vi "Diagnostics.vi"(10 "Parameters":variant, 11 "Process":refnum<class "Process.lvclass">) -> ()   [LabVIEW 2019, in "Diagnostics Addon Engine.lvlib"]
uses:
  Diagnostics Addon Engine.lvlib
  <vilib>/NI/NIVS Inline Async API/_VS Inline Async API/Process/Process.lvclass
  Addon Shared/Types/SysDef.Compile.ctl
  Addon Shared/Types/CAN.ctl
  Addon Shared/Types/CAN.Interface.ctl
  Addon Shared/Types/Protocol.ctl
  Addon Shared/Types/Transport.ctl
  Addon Shared/Types/986x.ctl
  Addon Shared/Types/Frame.Compile.ctl
  Addon Shared/Types/Type.ctl
  Addon Shared/Types/Signal.ctl
  Addon Shared/Types/DPID.ctl
  Addon Shared/Types/DPID.Rate.ctl
  Addon Shared/Types/DTC.Settings.ctl
  Addon Shared/Types/DTC.Descriptor.ctl
  Addon Shared/Types/Poll.Compiled.ctl
  Addon Shared/Types/Security.ctl
  Addon Shared/Types/Security.Type.ctl
  <vilib>/NI/NIVS Inline Async API/_Data Access Engine/Access Type Classes/Write/Write.lvclass/Write.ctl
  <vilib>/NI/NIVS Inline Async API/_Data Access Engine/Access Type Classes/ReadWrite/ReadWrite.lvclass/ReadWrite.ctl
  <vilib>/NI/NI VeriStand Addon Network Comm/Engine/VeriStand Comm.lvclass/VeriStand Comm.ctl
  <vilib>/NI/NIVS Inline Async API/_Data Access Engine/Access Type Classes/Read/Read.lvclass/Read.ctl
  <vilib>/NI/NIVS Inline Async API/_VS Inline Async API/Process/Process.lvclass/Process.ctl
  SubVIs/Frames.Refs.Cleanup.vi
  <vilib>/NI/NIVS Inline Async API/_Data Access Engine/Data Access Engine/Methods/Data.Processes.Execute.vi
  <vilib>/NI/NIVS Inline Async API/_Data Access Engine/Data Access Engine/Methods/Write.Data.vi
  <vilib>/NI/NI VeriStand Addon Network Comm/Engine/_SubVIs/Comm Connection Engine.vi
  <vilib>/NI/NI VeriStand Addon Network Comm/Engine/_SubVIs/Comm Command Engine.vi
  SubVIs/Diagnostics.Main.vi
  <vilib>/NI/NIVS Inline Async API/_VS Inline Async API/Process/Methods/Async.Processes.Report.vi
  <vilib>/NI/NI VeriStand Addon Network Comm/Engine/Comm API/Read Command.vi
  SubVIs/ServiceChannels.Status.Set.vi
  <vilib>/NI/NIVS Inline Async API/_Data Access Engine/Data Access Engine/Methods/ReadWrite.Data.Read.vi
  <vilib>/NI/NIVS Inline Async API/_Data Access Engine/Data Access Engine/Methods/ReadWrite.Data.Reset.vi
  <vilib>/NI/NI VeriStand Addon Network Comm/Engine/Comm API/Send Command.vi
  SubVIs/Commands.vi
  <vilib>/NI/NI VeriStand Addon Network Comm/Engine/Comm API/Send Commands.vi
  <vilib>/NI/NIVS Inline Async API/_Data Access Engine/Data Access Engine/Methods/Read.Data.vi
  SubVIs/DiagCANControl.WaitForFinish.vi
  <vilib>/NI/NIVS Inline Async API/_Data Access Engine/Access Type Classes/Write/Write.ProcessData.vi
  <vilib>/NI/STM/Connection Manager/TCP/Advanced/TCP Connection Manager (By Reference).vi
  <vilib>/Utility/error.llb/Clear Errors.vi
  <vilib>/NI/STM/Get Connection Reference.vi
  <vilib>/NI/STM/TCP/Get Connection Reference (TCP).vi
  <vilib>/NI/STM/Read Meta Data.vi
  <vilib>/NI/STM/TCP/Read Meta Data (TCP Ref).vi
  <vilib>/NI/AMC/Send Local Message.vi
  <vilib>/NI/Tools/Keyed Array/Add.vi
  <vilib>/NI/AMC/Read Next Message.vi
  <vilib>/NI/STM/Connection Manager/TCP/Advanced/TCP Check Connection (By Reference).vi
  SubVIs/Diagnostics.Main.UUDT.Engine.vi
  SubVIs/Diagnostics.Main.CmdResp.Engine.vi
  <vilib>/NI/NIVS Inline Async API/_VS Inline Async API/Error Handling Process/SubVIs/Error.ConvertArray.vi
  <vilib>/NI/Tools/Keyed Array/Index.vi
  <vilib>/NI/NIVS Inline Async API/_Data Access Engine/Data Access Engine/Methods/Write.Data.Buffer.vi
  Addon Shared/SubVIs/LookupID.Create.vi
  <vilib>/NI/NIVS Inline Async API/_Data Access Engine/Access Type Classes/ReadWrite/ReadWrite.ProcessData.Read.vi
  <vilib>/NI/NIVS Inline Async API/_Data Access Engine/Access Type Classes/ReadWrite/ReadWrite.ProcessData.Reset.vi
  Addon Shared/SubVIs/Format ECU Master Key to String.vi
  <vilib>/NI/AMC/Send Local Messages.vi
  <vilib>/NI/NIVS Inline Async API/_Data Access Engine/Access Type Classes/Read/Read.ProcessData.vi
  <vilib>/NI/NIVS Inline Async API/_Data Access Engine/Access Type Classes/Write/Write.Buffer.vi
  <vilib>/NI/NIVS Inline Async API/_Data Access Engine/Access Type Classes/Write/Write.Commit.vi
  <vilib>/NI/STM/SubVIs/Generate STM Error.vi
  <vilib>/NI/AMC/Create Single Message.vi
  <vilib>/NI/AMC/Update Message Routing Info.vi
  <vilib>/NI/Tools/Keyed Array/Map String.vi
  <vilib>/NI/AMC/Read Termination Message.vi
  SubVIs/Signals.Scale.EU.vi
  <vilib>/NI/NIVS Inline Async API/_Data Access Engine/Data Access Engine/Methods/Write.Data.Commit.vi
  Support Libraries/GMLAN/Utilities/Convert Data to DTCs.vi
  SubVIs/DTCs.List.Update.vi
  SubVIs/Restart.LocalStop.Read.vi
  Support Libraries/GMLAN/_SubVIs/ReadDiagnosticInformation_ByStatus.vi
  Support Libraries/GMLAN/_SubVIs/ReadDiagnosticInformation_sendOnChangeDTCCount.vi
  Support Libraries/GMLAN/_SubVIs/ReadFailureRecordData_readFailureRecordParameters.vi
  Support Libraries/GMLAN/_SubVIs/ReadDiagnosticInformation_readStatusOfDTCByDTCNumber.vi
  Support Libraries/GMLAN/GMLAN DynamicallyDefineMessage.vi
  SubVIs/Diagnostics.CheckTimeout.vi
  SubVIs/Status.Set.vi
  SubVIs/DPIDs.Find.vi
  Support Libraries/GMLAN/GMLAN ReadDataByPacketIdentifier.vi
  Support Libraries/GMLAN/GMLAN ReadDataByParameterIdentifier.vi
  SubVIs/Signals.Scale.Raw.vi
  Support Libraries/GMLAN/GMLAN DeviceControl.vi
  Support Libraries/GMLAN/GMLAN TesterPresent.vi
  Support Libraries/GMLAN/GMLAN InitiateDiagnosticOperation.vi
  Support Libraries/GMLAN/GMLAN DisableNormalCommunication.vi
  Support Libraries/GMLAN/GMLAN ReturnToNormalMode.vi
  SubVIs/ADCS.UnlockECUSecurity.vi
  <vilib>/NI/NI VeriStand Addon Network Comm/Engine/Comm API/Respond to Command.vi
  SubVIs/DTC.Descriptor.Override.vi
  Support Libraries/GMLAN/GMLAN ClearDiagnosticInformation.vi
  Support Libraries/GMLAN/GMLAN ReadDataByIdentifier.vi
  Support Libraries/GMLAN/GMLAN WriteDataByIdentifier.vi
  SubVIs/Frames.Lookup.Size.Get.vi
  SubVIs/ADCS.TesterPresent.vi
  <vilib>/NI/AMC/Create Multiple Messages.vi
  <vilib>/NI/Tools/String/Get Case Matching.vi
  Support Libraries/GMLAN/Utilities/Convert Raw Data to DTCs.vi
  Support Libraries/GMLAN/Utilities/GMLAN Service Broadcast.vi
  Support Libraries/GMLAN/GMLAN SecurityAccess.vi
  Support Libraries/GMLAN/_SubVIs/SecurityAccess_sendKey.vi
  SubVIs/Security.DLL.vi
  Support Libraries/GMLAN/_SubVIs/SecurityAccess_requestSeed.vi
  <vilib>/Automotive Diagnostic Command Set/Diagnostic Transport.llb/Diagnostic Service Send.vi
  <vilib>/Automotive Diagnostic Command Set/Diagnostic Transport.llb/Diagnostic Response Recv.vi
  <vilib>/Automotive Diagnostic Command Set/Diagnostic Transport.llb/ISOTP Transmit.vi
  <vilib>/Automotive Diagnostic Command Set/Diagnostic Transport.llb/ISOTP7 Transmit.vi
  <vilib>/Automotive Diagnostic Command Set/Diagnostic Transport.llb/DoIP Transmit.vi
  <vilib>/Automotive Diagnostic Command Set/Diagnostic Transport.llb/LIN ISOTP Transmit.vi
  <vilib>/Automotive Diagnostic Command Set/Diagnostic Transport.llb/Diagnostic Service Recv.vi
  <vilib>/Automotive Diagnostic Command Set/Diagnostic Transport.llb/ISOTP Send FF.vi
  <vilib>/Automotive Diagnostic Command Set/Diagnostic Transport.llb/ISOTP Send CFs.vi
  <vilib>/Automotive Diagnostic Command Set/Diagnostic Transport.llb/ISOTP Send Frame.vi
  <vilib>/Automotive Diagnostic Command Set/Diagnostic Transport.llb/ISOTP7 Send FF.vi
  <vilib>/Automotive Diagnostic Command Set/Diagnostic Transport.llb/ISOTP7 Send CFs.vi
  <vilib>/Automotive Diagnostic Command Set/Diagnostic Transport.llb/ISOTP7 Send Frame.vi
  <vilib>/Automotive Diagnostic Command Set/Diagnostic Transport.llb/DoIP TCP Msg Send.vi
  <vilib>/Automotive Diagnostic Command Set/Diagnostic Transport.llb/DoIP TCP Msg Recv.vi
  <vilib>/Automotive Diagnostic Command Set/Diagnostic Transport.llb/DoIP Check Addresses.vi
  <vilib>/Automotive Diagnostic Command Set/Diagnostic Transport.llb/DoIP Check ACK Code.vi
  <vilib>/Automotive Diagnostic Command Set/Diagnostic Transport.llb/ISOTP Receive.vi
  <vilib>/Automotive Diagnostic Command Set/Diagnostic Transport.llb/ISOTP7 Receive.vi
  <vilib>/Automotive Diagnostic Command Set/Diagnostic Transport.llb/DoIP Receive.vi
  <vilib>/Automotive Diagnostic Command Set/Diagnostic Transport.llb/LIN ISOTP Receive.vi
  <vilib>/Automotive Diagnostic Command Set/Diagnostic Transport.llb/Diag Get Globals.vi
  <vilib>/Automotive Diagnostic Command Set/Diagnostic Transport.llb/ISOTP Recv FC.vi
  <vilib>/Automotive Diagnostic Command Set/Diagnostic Transport.llb/ISOTP Send CF.vi
  <vilib>/Automotive Diagnostic Command Set/Diagnostic Transport.llb/Diag Fill Frame.vi
  <vilib>/Automotive Diagnostic Command Set/Diagnostic Transport.llb/ISOTP Calc Send Params.vi
  <vilib>/Automotive Diagnostic Command Set/Diagnostic Transport.llb/ISOTP7 Recv FC.vi
  <vilib>/Automotive Diagnostic Command Set/Diagnostic Transport.llb/ISOTP7 Send CF.vi
  <vilib>/Automotive Diagnostic Command Set/Diagnostic Transport.llb/DoIP Add Addresses.vi
  <vilib>/Automotive Diagnostic Command Set/Diagnostic Transport.llb/DoIP TCP Send.vi
  <vilib>/Automotive Diagnostic Command Set/Diagnostic Transport.llb/DoIP TCP Recv.vi
  <vilib>/Automotive Diagnostic Command Set/Diagnostic Transport.llb/DoIP Add Header.vi
  <vilib>/Automotive Diagnostic Command Set/Diagnostic Transport.llb/ISOTP Recv Frame.vi
  <vilib>/Automotive Diagnostic Command Set/Diagnostic Transport.llb/ISOTP Recv CFs.vi
  <vilib>/Automotive Diagnostic Command Set/Diagnostic Transport.llb/ISOTP7 Recv Frame.vi
  <vilib>/Automotive Diagnostic Command Set/Diagnostic Transport.llb/ISOTP7 Recv CFs.vi
  <vilib>/Automotive Diagnostic Command Set/Diagnostic Transport.llb/DoIP Send Alive.vi
  <vilib>/Automotive Diagnostic Command Set/Diagnostic Transport.llb/DoIP Check Error.vi
  <vilib>/Automotive Diagnostic Command Set/Diagnostic Transport.llb/ISOTP Check Redo.vi
  <vilib>/Automotive Diagnostic Command Set/Diagnostic Transport.llb/ISOTP Recv Block.vi
  <vilib>/Automotive Diagnostic Command Set/Diagnostic Transport.llb/ISOTP7 Recv Block.vi
  <vilib>/Automotive Diagnostic Command Set/Diagnostic Transport.llb/ISOTP Send FC.vi
  <vilib>/Automotive Diagnostic Command Set/Diagnostic Transport.llb/ISOTP Add CF.vi
  <vilib>/Automotive Diagnostic Command Set/Diagnostic Transport.llb/ISOTP7 Send FC.vi
  <vilib>/Automotive Diagnostic Command Set/Diagnostic Transport.llb/ISOTP7 Add CF.vi
  <vilib>/xnet/xnet.llb/XNET Clear.vi
  Addon Shared/SubVIs/Constants.vi
  <vilib>/xnet/xnet.llb/XNET Database Delete Object.vi
  <vilib>/xnet/xnet.llb/XNET Database Delete (Cluster).vi
  <vilib>/xnet/xnet.llb/XNET Database Close.vi
  <vilib>/xnet/xnet.llb/XNET Database Close (Database).vi
  <vilib>/Automotive Diagnostic Command Set/Diagnostic Transport.llb/Close Diagnostic.vi
  <vilib>/Utility/SystemLogging/Write to System Log.vi
  <vilib>/NI/AMC/Send Message.vi
  <vilib>/NI/NI VeriStand Addon Network Comm/Shared/Comm Constants.vi
  <vilib>/NI/AMC/Globals.vi
  SubVIs/CAN.Initialize.vi
  <vilib>/Automotive Diagnostic Command Set/Diagnostic Transport.llb/Diag Get Property.vi
  <vilib>/Automotive Diagnostic Command Set/Diagnostic Transport.llb/Diag Set Property.vi
  <vilib>/Automotive Diagnostic Command Set/Diagnostic Transport.llb/Diagnostic Service.vi
  <vilib>/Automotive Diagnostic Command Set/Diagnostic Transport.llb/Apply Success Failure Error.vi
  SubVIs/DPIDs.IDs.Sort.vi
  <vilib>/xnet/xnet.llb/XNET Convert.vi
  <vilib>/xnet/xnet.llb/XNET Convert (Frame CAN to Signal).vi
  <vilib>/xnet/xnet.llb/XNET Convert (Signal to Frame CAN).vi
  <vilib>/Automotive Diagnostic Command Set/Diagnostic Protocols.llb/TesterPresent.vi
  <vilib>/Automotive Diagnostic Command Set/Diagnostic Transport.llb/Diag Globals.vi
  <vilib>/Automotive Diagnostic Command Set/Diagnostic Transport.llb/CAN Send Frame Check Queue.vi
  <vilib>/Automotive Diagnostic Command Set/Diagnostic Transport.llb/Diag CAN get timestamp.vi
  <vilib>/Automotive Diagnostic Command Set/Diagnostic Transport.llb/Diag CAN read.vi
  <vilib>/Automotive Diagnostic Command Set/Diagnostic Transport.llb/ISOTP Calc Actual IO Mode.vi
  <vilib>/Automotive Diagnostic Command Set/Diagnostic Transport.llb/ISOTP Get FC Data.vi
  <vilib>/Automotive Diagnostic Command Set/Diagnostic Transport.llb/VWTP Write.vi
  <vilib>/Automotive Diagnostic Command Set/Diagnostic Transport.llb/DoIP Analyze Header.vi
  <vilib>/Automotive Diagnostic Command Set/Diagnostic Transport.llb/Diag CAN status.vi
  <vilib>/Automotive Diagnostic Command Set/Diagnostic Transport.llb/VWTP Read.vi
  <vilib>/Automotive Diagnostic Command Set/Diagnostic Transport.llb/Apply Diagnostic Error.vi
  <vilib>/Automotive Diagnostic Command Set/Diagnostic Protocols.llb/UDS TesterPresent.vi
  <vilib>/Automotive Diagnostic Command Set/Diagnostic Protocols.llb/UDS DiagnosticSessionControl.vi
  <vilib>/Automotive Diagnostic Command Set/Diagnostic Protocols.llb/StartDiagnosticSession.vi
  <vilib>/Automotive Diagnostic Command Set/Diagnostic Protocols.llb/StopDiagnosticSession.vi
  <vilib>/Automotive Diagnostic Command Set/Diagnostic Protocols.llb/UDS CommunicationControl.vi
  <vilib>/Automotive Diagnostic Command Set/Diagnostic Protocols.llb/DisableNormalMessageTransmission.vi
  <vilib>/Automotive Diagnostic Command Set/Diagnostic Protocols.llb/EnableNormalMessageTransmission.vi
  <vilib>/Automotive Diagnostic Command Set/Diagnostic Protocols.llb/UDS RequestSeed.vi
  <vilib>/Automotive Diagnostic Command Set/Diagnostic Protocols.llb/RequestSeed.vi
  <vilib>/Automotive Diagnostic Command Set/Diagnostic Protocols.llb/UDS SendKey.vi
  <vilib>/Automotive Diagnostic Command Set/Diagnostic Protocols.llb/SendKey.vi
  <vilib>/Automotive Diagnostic Command Set/Diagnostic Protocols.llb/UDS ReportDTCBySeverityMaskRecord.vi
  <vilib>/Automotive Diagnostic Command Set/Diagnostic Protocols.llb/UDS ReportSeverityInformationOfDTC.vi
  <vilib>/Automotive Diagnostic Command Set/Diagnostic Protocols.llb/UDS ReportDTCByStatusMask.vi
  <vilib>/Automotive Diagnostic Command Set/Diagnostic Protocols.llb/ReadStatusOfDTC.vi
  <vilib>/Automotive Diagnostic Command Set/Diagnostic Protocols.llb/ReadDTCByStatus.vi
  <vilib>/Automotive Diagnostic Command Set/Diagnostic Protocols.llb/ClearDiagnosticInformation.vi
  <vilib>/Automotive Diagnostic Command Set/Diagnostic Protocols.llb/UDS ClearDiagnosticInformation.vi
  <vilib>/Automotive Diagnostic Command Set/Diagnostic Protocols.llb/ReadDataByLocalIdentifier.vi
  <vilib>/Automotive Diagnostic Command Set/Diagnostic Protocols.llb/UDS ReadDataByIdentifier.vi
  <vilib>/Automotive Diagnostic Command Set/Diagnostic Protocols.llb/WriteDataByLocalIdentifier.vi
  <vilib>/Automotive Diagnostic Command Set/Diagnostic Protocols.llb/UDS WriteDataByIdentifier.vi
  <vilib>/Automotive Diagnostic Command Set/Diagnostic Protocols.llb/UDS ControlDTCSetting.vi
  <vilib>/Automotive Diagnostic Command Set/Diagnostic Protocols.llb/ControlDTCSetting.vi
  <vilib>/Automotive Diagnostic Command Set/Diagnostic Protocols.llb/ECUReset.vi
  <vilib>/Automotive Diagnostic Command Set/Diagnostic Protocols.llb/UDS ECUReset.vi
  <vilib>/Automotive Diagnostic Command Set/Diagnostic Protocols.llb/ReadMemoryByAddress.vi
  <vilib>/Automotive Diagnostic Command Set/Diagnostic Protocols.llb/UDS06 ReadMemoryByAddress.vi
  <vilib>/Automotive Diagnostic Command Set/Diagnostic Protocols.llb/UDS ReadMemoryByAddress.vi
  <vilib>/Automotive Diagnostic Command Set/Diagnostic Protocols.llb/WriteMemoryByAddress.vi
  <vilib>/Automotive Diagnostic Command Set/Diagnostic Protocols.llb/UDS06 WriteMemoryByAddress.vi
  <vilib>/Automotive Diagnostic Command Set/Diagnostic Protocols.llb/UDS WriteMemoryByAddress.vi
  <vilib>/Automotive Diagnostic Command Set/Diagnostic Protocols.llb/InputOutputControlByLocalIdentifier.vi
  <vilib>/Automotive Diagnostic Command Set/Diagnostic Protocols.llb/UDS InputOutputControlByIdentifier.vi
  <vilib>/Automotive Diagnostic Command Set/Diagnostic Protocols.llb/StartRoutineByLocalIdentifier.vi
  <vilib>/Automotive Diagnostic Command Set/Diagnostic Protocols.llb/UDS RoutineControl.vi
  <vilib>/Automotive Diagnostic Command Set/Diagnostic Protocols.llb/RequestRoutineResultsByLocalIdentifier.vi
  <vilib>/Automotive Diagnostic Command Set/Diagnostic Protocols.llb/StopRoutineByLocalIdentifier.vi
  <vilib>/xnet/xnet.llb/XNET Read.vi
  <vilib>/xnet/xnet.llb/XNET Read (Frame CAN).vi
  <vilib>/Automotive Diagnostic Command Set/Diagnostic Protocols.llb/Convert to Phys.vi
  <vilib>/NI/STM/Read Message.vi
  <vilib>/NI/STM/TCP/Read Message (TCP).vi
  <vilib>/NI/AMC/Create Message Queue.vi
  <vilib>/NI/STM/Write Message.vi
  <vilib>/NI/STM/TCP/Write Message (TCP).vi
  <vilib>/NI/AMC/Destroy Message Queue.vi
  <vilib>/NI/STM/TCP/Read Meta Data (TCP Clst).vi
  Addon Shared/Diagnostics Addon Shared.lvlib
  <vilib>/NI/NI VeriStand Addon Network Comm/Engine/VeriStand Comm.lvclass
panel:
  in  "Error":errorcluster
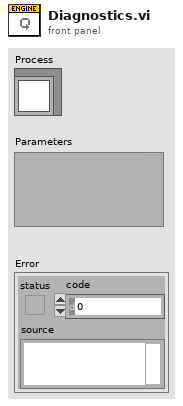
[diagram p1: front panel]
types:
  T1 = typedef "Diagnostics Addon Shared.lvlib/SysDef.Compile.ctl" = cluster{"Name":string, "CAN":T2, "986x":T6, "Reads":T7[], "Frames Lookup":variant, "Writes":T7[], "DPIDs":T10[], "DPID Lookup":variant, "DTC":T12, "Created DTCs":u32, "Polls":T14[], "Service Channels Status Lookup":variant, "Trigger Lookup":variant, "Security":T15}
  T2 = typedef "Diagnostics Addon Shared.lvlib/CAN.ctl" = cluster{"Interface":T3, "Baud Rate":u64, "Diagnostic Protocol":T4, "Transport Protocol":T5, "Transmit ID":u32, "Receive ID":u32, "Transmit Extension":u8, "Receive Extension":u8, "Receive UUDT ID":u32, "Enable Stream":bool, "VW TP Channel ID":u32, "Fill Frame":bool, "Fill Byte":u8, "Termination":bool, "LIN Cluster":refnum<k21>, "NAD":u8, "IO Mode":u32, "Max DLC":u16, "FD Baud Rate":u64, "Timeout":u32}
  T3 = typedef "Diagnostics Addon Shared.lvlib/CAN.Interface.ctl" = string
  T4 = typedef "Diagnostics Addon Shared.lvlib/Protocol.ctl" = enum16{"GMLAN", "KWP-2000", "UDS", "User-Defined"}
  T5 = typedef "Diagnostics Addon Shared.lvlib/Transport.ctl" = enum16{"ISO TP - Normal Mode", "ISO TP - Mixed Mode", "VW TP 2.0", "Diagnostics on IP", "ISO TP LIN"}
  T6 = typedef "Diagnostics Addon Shared.lvlib/986x.ctl" = cluster{"Enable":bool, "RIO Device":string, "Bitfile":path}
  T7 = typedef "Diagnostics Addon Shared.lvlib/Frame.Compile.ctl" = cluster{"ID":u32, "Type":T8, "Signals":T9[]}
  T8 = typedef "Diagnostics Addon Shared.lvlib/Type.ctl" = enum16{"DID", "CDID", "PID", "CPID", "Read Memory", "Write Memory", "IO Control", "Routine Start", "Routine Request", "Routine Stop", "User Defined", "DTC Control", "Clear DTCs", "Read DTCs", "Start DTCs", "DTC Change Count", "Tester Present", "Unlock ECU", "Reset ECU", "Diag Session Control", "Communication Control", "DPID Control", "Poll Control", "Diag CAN Control"}
  T9 = typedef "Diagnostics Addon Shared.lvlib/Signal.ctl" = cluster{"Start Bit":u32, "Length":u32, "Scaling Factor":dbl, "Scaling Offset":dbl, "Minimum":dbl, "Maximum":dbl, "Data Type":u32, "Byte Order":u32, "Default Value":dbl, "Name":string, "Units":string}
  T10 = typedef "Diagnostics Addon Shared.lvlib/DPID.ctl" = cluster{"DPID ID":u8, "Speed":T11, "PIDs":u16[]}
  T11 = typedef "Diagnostics Addon Shared.lvlib/DPID.Rate.ctl" = enum16{"Slow", "Medium", "Fast"}
  T12 = typedef "Diagnostics Addon Shared.lvlib/DTC.Settings.ctl" = cluster{"Descriptor":T13, "Value.Code":dbl[], "Value.String":string[], "Value.J2012String":string[], "Status.Code":dbl[], "Status.String":string[]}
  T13 = typedef "Diagnostics Addon Shared.lvlib/DTC.Descriptor.ctl" = cluster{"DTC Byte Length":i32, "Status Byte Length":i32, "Add Data Byte Length":i32, "Byte Order":enum16{"Motorola", "Intel"}}
  T14 = typedef "Diagnostics Addon Shared.lvlib/Poll.Compiled.ctl" = cluster{"Speed":T11, "DID IDs":u32[], "PID IDs":u32[]}
  T15 = typedef "Diagnostics Addon Shared.lvlib/Security.ctl" = cluster{"Type":T16, "Source DLL Path":path, "Target DLL Path":path, "Security Level":u8}
  T16 = typedef "Diagnostics Addon Shared.lvlib/Security.Type.ctl" = enum16{"None", "DLL", "MasterKey"}
  T17 = typedef "Diagnostics Addon Engine.lvlib/Diagnostics.State.ctl" = cluster{"Comm":refnum<class "VeriStand Comm.lvclass">, "Parameters":T1, "ADCS Connection":T18, "XNET References":T23, "XNETEngine (GMLAN)":T24, "Process":refnum<class "Process.lvclass">, "Reads":T25, "Writes":T26, "Cmds":T27, "DTCs":T25, "DTC Count":T25, "Status":T25, "Triggers":T27, "CANConnected":T25, "LocalStop":refnum<data-value>, "LocalCommStatus":refnum<data-value>, "Service Channels Status":T25, "Settings":T26}
  T18 = typedef "NI_Automotive Diagnostic Command Set.lvlib/Diag Reference.ctl" = cluster{"Diag CAN Handle":u32, "Transport Protocol":T19, "Receive Address Extension":u8, "Transmit Address Extension":u8, "Receive CAN Id":u32, "Transmit CAN Id":u32, "Log Frames ?":bool, "My TP Address":u8, "Other TP Address":u8, "T1":u16, "T2":u16, "T3":u16, "T4":u16, "Tx SN":u8, "Block Size":u8, "Rx SN":u8, "VW TP Initialized?":bool, "Tx block no":u8, "baud rate":u64, "Interface":string, "Channel Diag CAN Handle":u32, "UDP Connection ID":refnum<k16>, "TCP Connection ID":refnum<k5>, "Target IP Addr":u32, "Source Address":u16, "Target Address":u16, "Send Header NACK?":bool, "DLL Handle":u32, "NAD":u8, "Time Stamp read first":dbl, "Time Stamp read last":dbl, "Time Stamp write first":dbl, "Time Stamp write last":dbl, "Time Stamp write":dbl, "Time Stamp read":dbl, " I/O Mode":u32, "FD Baudrate":u64, "TX_DL":u16, "RX_DL":u16, "DoIP Protocol Version":T20, " Selected I/O Mode":u32, "TesterPresent Counter":u32, "TesterPresent Limit":u32, "TesterPresent Tick[ms]":i32, "TesterPresent RequireResponse?":bool, "TesterPresent Stored Ref?":bool, "TesterPresent Message":u8[], "TesterPresent Task Handle":i32, "TesterPresent Semaphore":T21, "Response Plausibility Check":u32, "Default Version?":bool, "Diagostic Globals":T22, "Session-based Properties?":bool}
  T19 = typedef "NI_Automotive Diagnostic Command Set.lvlib/Transport Protocol Selector.ctl" = enum16{"ISO TP - Normal Mode", "ISO TP - Mixed Mode", "VW TP 2.0", "Diagnostics on IP", "ISO TP LIN"}
  T20 = typedef "NI_Automotive Diagnostic Command Set.lvlib/DoIP Protocol Version.ctl" = u8
  T21 = typedef "Semaphore RefNum" = refnum<k1>
  T22 = typedef "NI_Automotive Diagnostic Command Set.lvlib/Diag Globals.ctl" = cluster{"Timeout FC (Bs)":u32, "Timeout CF (Cr)":u32, "Timeout Diag Command":u32, "Receive Block Size (BS)":u8, "Wait Time CF (STmin)":u8, "Max Waits (N_WFTmax)":u8, "Waits to Send (N_WAIT)":i32, "Time between Waits (TW)":u32, "Fill CAN Frames?":bool, "Fill Byte":u32, "Invalid Response as Error?":bool, "Max RspPending Count":u32, "VWTP Command Timeout":u32, "Transport Protocol":T19, "Diag CAN Handle":u32, "DLL Handle":u32, "Timeout RspPending":u32}
  T23 = typedef "Diagnostics Addon Engine.lvlib/XNET.Refs.ctl" = cluster{"Database":refnum<k21>, "GMLAN DPID Session":refnum<k21>, "Cluster":refnum<k21>}
  T24 = typedef "AMC.lvlib/Message Queue.ctl" = refnum<queue>
  T25 = typedef "Data Access Engine.lvlib/Data Access Engine.lvclass/Write.DVR.ctl" = refnum<data-value>
  T26 = typedef "Data Access Engine.lvlib/Data Access Engine.lvclass/Read.DVR.ctl" = refnum<data-value>
  T27 = typedef "Data Access Engine.lvlib/Data Access Engine.lvclass/ReadWrite.DVR.ctl" = refnum<data-value>
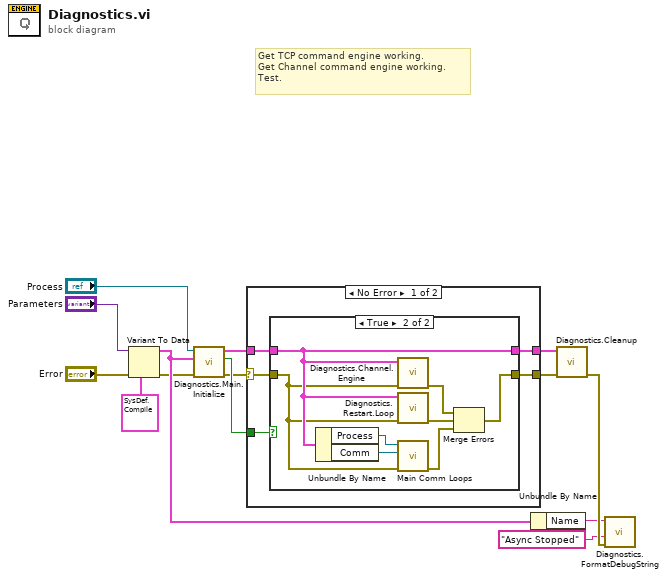
[diagram p0: block diagram]
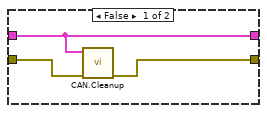
[diagram p2: hidden frame]
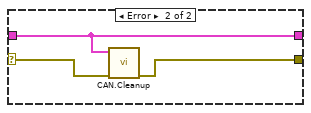
[diagram p3: hidden frame]
diagram:
  # "Get TCP command engine working.\nGet Channel command engine working.\nTest."
  n1 = Variant To Data(error in="Error", type=T1 {"Name"="", "CAN"={"Interface"="", "Baud Rate"=0, "Diagnostic Protocol"=enum."GMLAN", "Transport Protocol"=enum."ISO TP - Normal Mode", "Transmit ID"=0, "Receive ID"=2, "Transmit Extension"=1, "Receive Extension"=255, "Receive UUDT ID"=0, "Enable Stream"=TRUE, "VW TP Channel ID"=1, "Fill Frame"=FALSE, "Fill Byte"=0, "Termination"=FALSE, "LIN Cluster"="", "NAD"=8, "IO Mode"=0, "Max DLC"=0, "FD Baud Rate"=2, "Timeout"=1}, "986x"={"Enable"=FALSE, "RIO Device"="", "Bitfile"=path ""}, "Reads"=[], "Frames Lookup"=variant(enum16{"GMLAN", "KWP-2000", "UDS"} enum."GMLAN"), "Writes"=[], "DPIDs"=[], "DPID Lookup"=variant(u32 0), "DTC"={"Descriptor"={"DTC Byte Length"=1, "Status Byte Length"=1, "Add Data Byte Length"=1, "Byte Order"=enum."Motorola"}, "Value.Code"=[], "Value.String"=[], "Value.J2012String"=[], "Status.Code"=[], "Status.String"=[]}, "Created DTCs"=0, "Polls"=[], "Service Channels Status Lookup"=variant, "Trigger Lookup"=variant, "Security"={"Type"=enum."None", "Source DLL Path"=path "", "Target DLL Path"=path "", "Security Level"=0}} ("VS Main Configuration"), Variant="Parameters") -> (data=w4:T1, error out=w3:errorcluster)
  n2 = call "Diagnostics.Main.Initialize.vi"("error in (no error)"=w3, "Parameters"=w4, "Process"="Process") -> ("error out"=w8:errorcluster, "Execute"=w9:bool, "State Variables Out"=w10:T17)  [unwired: 6 in]
  n3 = case shown="No Error" w8 {
    selector: w8 -> [w15 w32]
    tunnel: [w19 w31] -> w14
    tunnel: [w18 w33] -> w5
    tunnel: w10 -> [w17 w33]
    tunnel: w9 -> [w16 _]
    frame No Error {
      n4 = case shown="True" w16 {
        tunnel: [w20 w30] -> w19
        tunnel: [w22 w25] -> w18
        tunnel: w15 -> [w21 w23]
        tunnel: w17 -> [w22 w25]
        frame False {
          n5 = call "CAN.Cleanup.vi"("error in (no error)"=w21, "State Variables Out"=w22) -> ("error out"=w20:errorcluster)  [unwired: 9 in]
        }
        frame True {
          n6 = Unbundle By Name(w25) -> ("Process"=w27:refnum<class "Process.lvclass">, "Comm"=w28:refnum<class "VeriStand Comm.lvclass">)
          n7 = call "Diagnostics.Channel.Engine.vi"("error in"=w23, "State Variables"=w25) -> ("error out"=w24:errorcluster)  [unwired: 9 in]
          n8 = call "Diagnostics.Restart.Loop.vi"("error in (no error)"=w23, "State Variables Out"=w25) -> ("Error Out"=w29:errorcluster)  [unwired: 9 in]
          n9 = call <vilib>:"Main Comm Loops.vi"("error in (no error)"=w23, "Comm.lvclass"=w28, "Process"=w27) -> ("error out"=w26:errorcluster)  [unwired: 8 in]
          n10 = Merge Errors(w24, w29, w26) -> (w30:errorcluster)
        }
      }
    }
    frame Error {
      n11 = call "CAN.Cleanup.vi"("error in (no error)"=w32, "State Variables Out"=w33) -> ("error out"=w31:errorcluster)  [unwired: 9 in]
    }
  }
  n12 = Unbundle By Name(w4) -> ("Name"=w2:string)
  n13 = call "Diagnostics.Cleanup.vi"("error in (no error)"=w14, "State Variables"=w5) -> ("error out"=w13:errorcluster)  [unwired: 9 in]
  n14 = call "Diagnostics.FormatDebugString.vi"("error in (no error)"=w13, "State"="Async Stopped" ("string"), "Name"=w2) -> ()  [unwired: 8 in, 1 out]
